vi "MLP.vi"() -> ()   [LabVIEW 2015]
uses:
  <vilib>/Analysis/baseanly.llb/Real A x B.vi
  <vilib>/Analysis/NI_AALBase.lvlib
panel:
  out "Image Classes":i32[](array[numeric])
  out "Character Images":picture[](array[picture])
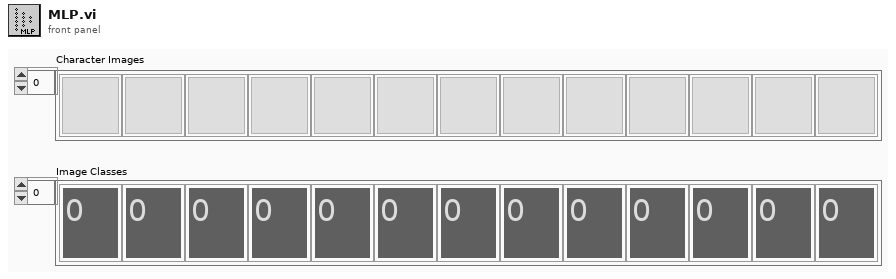
[diagram p1: front panel]
types:
  T1 = typedef "NI_Matrix.lvlib/RealMatrix.ctl" = dbl[][]
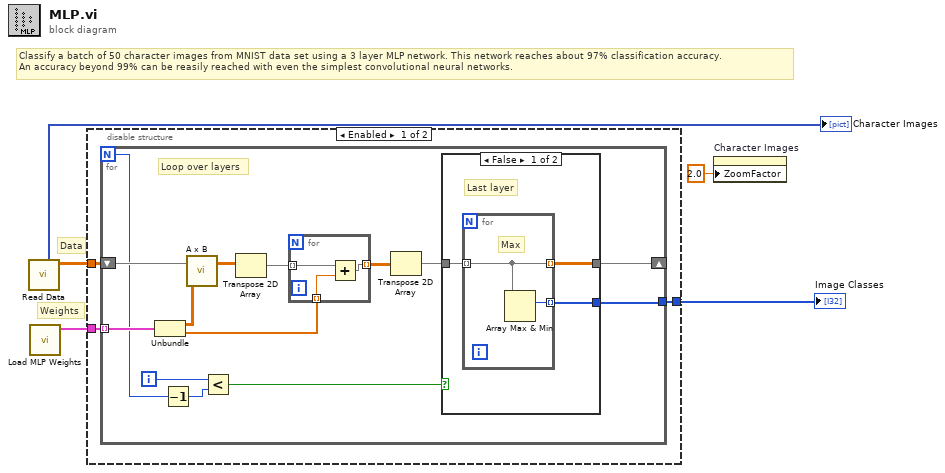
[diagram p0: block diagram]
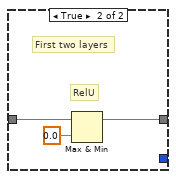
[diagram p2: hidden frame]
diagram:
  # "Data"
  # "Weights"
  # "Classify a batch of 50 character images from MNIST data set using a 3 layer MLP network. This network reaches about 97% classification accuracy.\nAn accuracy beyond 99% can be reasily reached with even the simplest convolutional neural networks."
  n1 = call "Read Data.vi"() -> ("Normalized Data"=w2:dbl[][], "Character Images"=→"Character Images":picture[])  [unwired: 9 in, 1 out]
  n2 = call "Load MLP Weights.vi"() -> ("Weights"=w5:cluster{"Weights":dbl[][], "Biases":dbl[]}[])  [unwired: 10 in, 1 out]
  n3 = disable-structure shown="Enabled" {
    disable-tunnel: w5 -> [w8 _]
    disable-tunnel: [w7 _] -> w3
    disable-tunnel: w2 -> [w6 _]
    frame Enabled {
      n4 = for {
        N -> [w18]
        tunnel: w8 -> [w20] mode=indexing
        shift-right: [w21] -> _
        shift-left: w6 -> [w22]
        tunnel: [w14] -> w7
        i -> [w16]
        # "Loop over layers"
        n5 = Unbundle(w20) -> ("Weights"=w19:dbl[][], "Biases"=w9:dbl[])
        n6 = Decrement(x=w18) -> (x-1=w15:i32)
        n7 = call-poly <vilib>:"A x B.vi"("B"=w19, "A"=w22) -> ("A x B"=w12:T1)  [unwired: 1 out]
        n8 = Less?(x=w16, y=w15) -> (x < y?=w17:bool)
        n9 = Transpose 2D Array(2D array=w12) -> (transposed array=w13:T1)
        n10 = for {
          tunnel: [w33] -> w11 mode=indexing
          tunnel: w13 -> [w32] mode=indexing
          tunnel: w9 -> [w31] mode=indexing
          n11 = Add ("Add.vi")(x=w32, y=w31) -> (x+y=w33:dbl[])
        }
        n12 = Transpose 2D Array(2D array=w11) -> (transposed array=w10:dbl[][])
        n13 = case shown="False" w17 {
          tunnel: w10 -> [w25 w29]
          tunnel: [w23 w28] -> w21
          tunnel: [w24 _] -> w14
          frame False {
            # "Last layer"
            n14 = for {
              tunnel: w25 -> [w26] mode=indexing
              tunnel: [w27] -> w24 mode=indexing
              tunnel: [w26] -> w23 mode=indexing
              # "Max"
              n15 = Array Max & Min(array=w26) -> (max index (indices)=w27:i32)  [unwired: 3 out]
            }
          }
          frame True {
            # "First two layers"
            # "RelU"
            n16 = Max & Min(x=w29, y=0.0 ("f")) -> (max(x,y)=w28:dbl[][])  [unwired: 1 out]
          }
        }
      }
    }
    frame Disabled {
    }
  }
  "Image Classes" <- w3
  n17 = property on="Character Images" class="Pict"("ZoomFactor"=sgl 2.0 ("Zoom Factor")) -> ()  [unwired: 2 in, 2 out]
